vi "Rang wear off.vi"(8 "error in (no error)":errorcluster caption="错误输入（无错误）", 11 "Popup 输入":refnum<class "Popup.lvclass"> caption="DNL_LabVIEW Object in") -> (0 "error out":errorcluster caption="错误输出", 3 "Popup 输出":refnum<class "Popup.lvclass"> caption="DNL_LabVIEW Object out")   [LabVIEW 2017, in "Popup.lvclass"]
uses:
  Popup.lvclass
  Popup.lvclass/Popup.ctl
  <vilib>/Utility/Data Type/NI_Data Type.lvlib
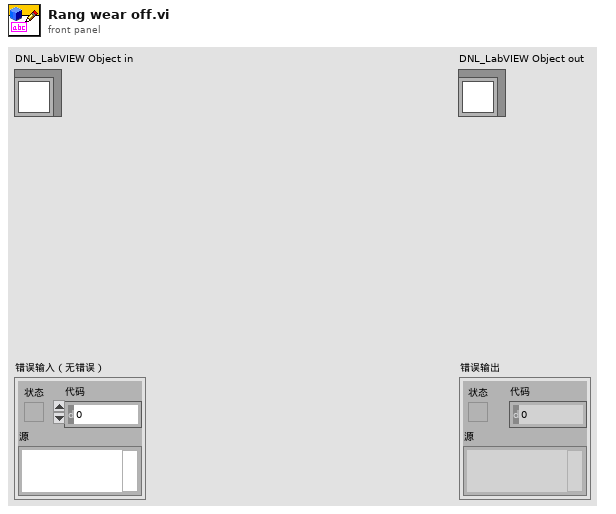
[diagram p1: front panel]
types:
  T1 = typedef "NI_Data Type.lvlib/Data Type.ctl" = enum8{"Invalid Type", "Void", "I8", "I16", "I32", "I64", "U8", "U16", "U32", "U64", "Single Float", "Double Float", "Extended Float", "Single Complex", "Double Complex", "Extended Complex", "Enum U8", "Enum U16", "Enum U32", "Enum U64", "Single Float With Unit", "Double Float With Unit", "Extended Float With Unit", "Single Complex with Unit", "Double Complex with Unit", "Extended Complex with Unit", "Boolean", "String", "Path", "Picture", "Tag", "Array", "Cluster", "Variant", "LV Variant", "Waveform", "Timestamp", "Digital Waveform", "Digital Data", "ExpressData", "Refnum", "External Data", "VI", "Poly VI", "LabVIEW Class Instance", "Fixed Point"}
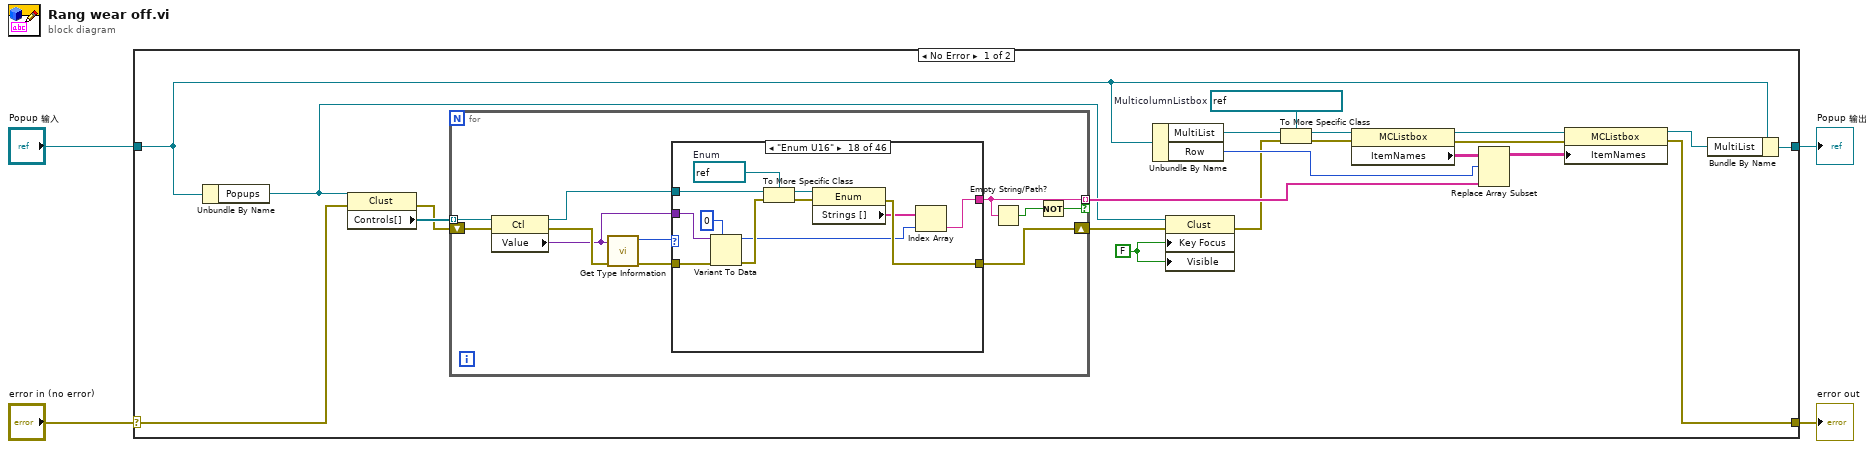
[diagram p0: block diagram]
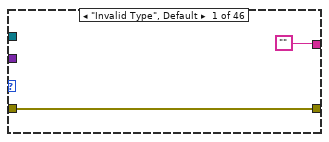
[diagram p2: hidden frame]
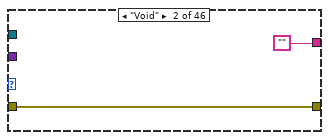
[diagram p3: hidden frame]
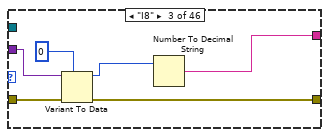
[diagram p4: hidden frame]
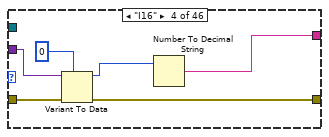
[diagram p5: hidden frame]
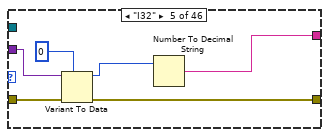
[diagram p6: hidden frame]
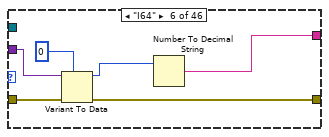
[diagram p7: hidden frame]
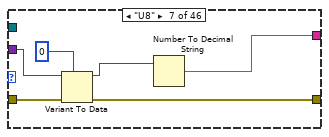
[diagram p8: hidden frame]
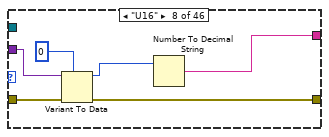
[diagram p9: hidden frame]
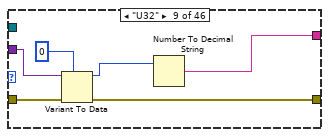
[diagram p10: hidden frame]
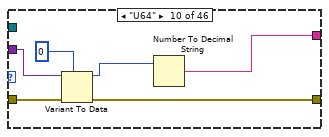
[diagram p11: hidden frame]
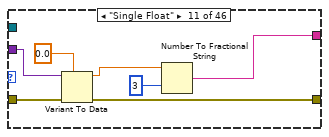
[diagram p12: hidden frame]
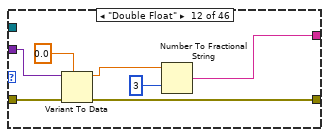
[diagram p13: hidden frame]
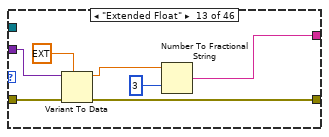
[diagram p14: hidden frame]
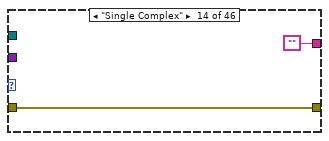
[diagram p15: hidden frame]
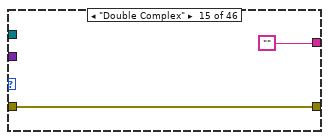
[diagram p16: hidden frame]
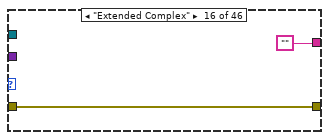
[diagram p17: hidden frame]
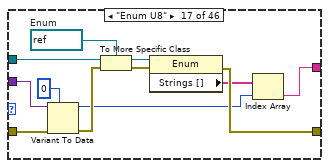
[diagram p18: hidden frame]
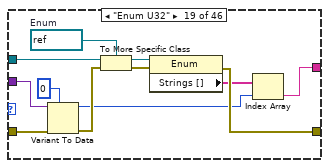
[diagram p19: hidden frame]
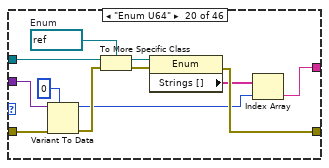
[diagram p20: hidden frame]
diagram:
  n1 = case shown="No Error" "error in (no error)" {
    selector: "error in (no error)" -> [w25 w230]
    tunnel: [w9 w230] -> w3
    tunnel: [w22 w229] -> w1
    tunnel: "Popup 输入" -> [w21 w229]
    frame No Error {
      w6 = FALSE
      w17 = refnum<vi> refnum  # MulticolumnListbox
      n2 = Unbundle By Name(w21) -> ("Popups"=w7:refnum<vi>)
      n3 = property class="Clust"(reference=w7, error in=w25) -> (error out=w23:errorcluster, "Controls[]"=w24:refnum<vi>[])  [unwired: 1 out]
      n4 = for {
        tunnel: w24 -> [w36] mode=indexing
        shift-right: [w30] -> w8
        shift-left: w23 -> [w35]
        tunnel: [w27] -> w14 mode=indexing if=w26
        n5 = property class="Ctl"(reference=w36, error in=w35) -> (reference out=w29:refnum<vi>, error out=w33:errorcluster, "Value"=w31:variant)
        n6 = call <vilib>:"Get Type Information.vi"("error in (no error)"=w33, "Variant"=w31) -> ("error out"=w32:errorcluster, "Type"=w34:T1)  [unwired: 5 in, 3 out]
        n7 = case shown="\"Enum U16\"" w34 {
          tunnel: w32 -> [w38 w40 w45 w51 w57 w63 w69 w75 w81 w87 w95 w102 w109 w111 w112 w114 w125 w137 w149 w161 w164 w166 w168 w170 w172 w174 w183 w188 w194 w196 w198 w200 w202 w204 w206 w208 w210 w212 w214 w216 w218 w220 w222 w224 w226 w228]
          tunnel: w31 -> [_ _ w46 w52 w58 w64 w70 w76 w82 w88 w94 w101 w108 _ _ _ w126 w138 w150 w162 _ _ _ _ _ _ w182 w187 w193 _ _ _ _ _ _ _ _ _ _ _ _ _ _ _ _ _]
          tunnel: [w38 w40 w43 w49 w55 w61 w67 w73 w79 w85 w92 w99 w106 w111 w112 w114 w119 w131 w143 w155 w164 w166 w168 w170 w172 w174 w176 w185 w190 w196 w198 w200 w202 w204 w206 w208 w210 w212 w214 w216 w218 w220 w222 w224 w226 w228] -> w30
          tunnel: ["" "" w41 w47 w53 w59 w65 w71 w77 w83 w89 w96 w103 "" "" "" w116 w128 w140 w152 "" "" "" "" "" "" w177 w184 w189 "" "" "" "" "" "" "" "" "" "" "" "" "" "" "" "" ""] -> w27
          tunnel: w29 -> [_ _ _ _ _ _ _ _ _ _ _ _ _ _ _ _ w127 w139 w151 w163 _ _ _ _ _ _ _ _ _ _ _ _ _ _ _ _ _ _ _ _ _ _ _ _ _ _]
          frame "Invalid Type", Default {
          }
          frame "Void" {
          }
          frame "I8" {
            n8 = Variant To Data(error in=w45, type=i8 0, Variant=w46) -> (data=w42:i8, error out=w43:errorcluster)
            n9 = Number To Decimal String(number=w42) -> (decimal integer string=w41:string)  [unwired: 1 in]
          }
          frame "I16" {
            n10 = Variant To Data(error in=w51, type=i16 0, Variant=w52) -> (data=w48:i16, error out=w49:errorcluster)
            n11 = Number To Decimal String(number=w48) -> (decimal integer string=w47:string)  [unwired: 1 in]
          }
          frame "I32" {
            n12 = Variant To Data(error in=w57, type=0, Variant=w58) -> (data=w54:i32, error out=w55:errorcluster)
            n13 = Number To Decimal String(number=w54) -> (decimal integer string=w53:string)  [unwired: 1 in]
          }
          frame "I64" {
            n14 = Variant To Data(error in=w63, type=i64 0, Variant=w64) -> (data=w60:i64, error out=w61:errorcluster)
            n15 = Number To Decimal String(number=w60) -> (decimal integer string=w59:string)  [unwired: 1 in]
          }
          frame "U8" {
            n16 = Variant To Data(error in=w69, type=u8 0, Variant=w70) -> (data=w66:u8, error out=w67:errorcluster)
            n17 = Number To Decimal String(number=w66) -> (decimal integer string=w65:string)  [unwired: 1 in]
          }
          frame "U16" {
            n18 = Variant To Data(error in=w75, type=u16 0, Variant=w76) -> (data=w72:u16, error out=w73:errorcluster)
            n19 = Number To Decimal String(number=w72) -> (decimal integer string=w71:string)  [unwired: 1 in]
          }
          frame "U32" {
            n20 = Variant To Data(error in=w81, type=u32 0, Variant=w82) -> (data=w78:u32, error out=w79:errorcluster)
            n21 = Number To Decimal String(number=w78) -> (decimal integer string=w77:string)  [unwired: 1 in]
          }
          frame "U64" {
            n22 = Variant To Data(error in=w87, type=u64 0, Variant=w88) -> (data=w84:u64, error out=w85:errorcluster)
            n23 = Number To Decimal String(number=w84) -> (decimal integer string=w83:string)  [unwired: 1 in]
          }
          frame "Single Float" {
            n24 = Variant To Data(error in=w95, type=sgl 0.0, Variant=w94) -> (data=w91:sgl, error out=w92:errorcluster)
            n25 = Number To Fractional String(number=w91, precision (6)=3) -> (F-format string=w89:string)  [unwired: 2 in]
          }
          frame "Double Float" {
            n26 = Variant To Data(error in=w102, type=0.0, Variant=w101) -> (data=w98:dbl, error out=w99:errorcluster)
            n27 = Number To Fractional String(number=w98, precision (6)=3) -> (F-format string=w96:string)  [unwired: 2 in]
          }
          frame "Extended Float" {
            n28 = Variant To Data(error in=w109, type=ext 0.0, Variant=w108) -> (data=w105:ext, error out=w106:errorcluster)
            n29 = Number To Fractional String(number=w105, precision (6)=3) -> (F-format string=w103:string)  [unwired: 2 in]
          }
          frame "Single Complex" {
          }
          frame "Double Complex" {
          }
          frame "Extended Complex" {
          }
          frame "Enum U8" {
            w122 = refnum<vi> refnum  # Enum
            n30 = Variant To Data(error in=w125, type=u8 0, Variant=w126) -> (data=w117:u8, error out=w123:errorcluster)
            n31 = To More Specific Class(target class=w122, reference=w127, error in=w123) -> (specific class reference=w121:refnum<vi>, error out=w120:errorcluster)
            n32 = property class="Enum"(reference=w121, error in=w120) -> (error out=w119:errorcluster, "Strings []"=w118:string[])  [unwired: 1 out]
            n33 = Index Array(array=w118, index=w117) -> (element=w116:string)
          }
          frame "Enum U16" {
            w134 = refnum<vi> refnum  # Enum
            n34 = Variant To Data(error in=w137, type=u16 0, Variant=w138) -> (data=w129:u16, error out=w135:errorcluster)
            n35 = To More Specific Class(target class=w134, reference=w139, error in=w135) -> (specific class reference=w133:refnum<vi>, error out=w132:errorcluster)
            n36 = property class="Enum"(reference=w133, error in=w132) -> (error out=w131:errorcluster, "Strings []"=w130:string[])  [unwired: 1 out]
            n37 = Index Array(array=w130, index=w129) -> (element=w128:string)
          }
          frame "Enum U32" {
            w146 = refnum<vi> refnum  # Enum
            n38 = Variant To Data(error in=w149, type=u32 0, Variant=w150) -> (data=w141:u32, error out=w147:errorcluster)
            n39 = To More Specific Class(target class=w146, reference=w151, error in=w147) -> (specific class reference=w145:refnum<vi>, error out=w144:errorcluster)
            n40 = property class="Enum"(reference=w145, error in=w144) -> (error out=w143:errorcluster, "Strings []"=w142:string[])  [unwired: 1 out]
            n41 = Index Array(array=w142, index=w141) -> (element=w140:string)
          }
          frame "Enum U64" {
            w158 = refnum<vi> refnum  # Enum
            n42 = Variant To Data(error in=w161, type=u64 0, Variant=w162) -> (data=w153:u64, error out=w159:errorcluster)
            n43 = To More Specific Class(target class=w158, reference=w163, error in=w159) -> (specific class reference=w157:refnum<vi>, error out=w156:errorcluster)
            n44 = property class="Enum"(reference=w157, error in=w156) -> (error out=w155:errorcluster, "Strings []"=w154:string[])  [unwired: 1 out]
            n45 = Index Array(array=w154, index=w153) -> (element=w152:string)
          }
          frame "Single Float With Unit" {
          }
          frame "Double Float With Unit" {
          }
          frame "Extended Float With Unit" {
          }
          frame "Single Complex with Unit" {
          }
          frame "Double Complex with Unit" {
          }
          frame "Extended Complex with Unit" {
          }
          frame "Boolean" {
            n46 = Variant To Data(error in=w183, type=FALSE, Variant=w182) -> (data=w180:bool, error out=w176:errorcluster)
            n47 = Select(t="TURE", s=w180, f="FALES") -> (s? t:f=w177:string)
          }
          frame "String" {
            n48 = Variant To Data(error in=w188, type="", Variant=w187) -> (data=w184:string, error out=w185:errorcluster)
          }
          frame "Path" {
            n49 = Variant To Data(error in=w194, type=path "", Variant=w193) -> (data=w191:path, error out=w190:errorcluster)
            n50 = Path To String(path=w191) -> (string=w189:string)
          }
          frame "Picture" {
          }
          frame "Tag" {
          }
          frame "Array" {
          }
          frame "Cluster" {
          }
          frame "Variant" {
          }
          frame "LV Variant" {
          }
          frame "Waveform" {
          }
          frame "Timestamp" {
          }
          frame "Digital Waveform" {
          }
          frame "Digital Data" {
          }
          frame "ExpressData" {
          }
          frame "Refnum" {
          }
          frame "External Data" {
          }
          frame "VI" {
          }
          frame "Poly VI" {
          }
          frame "LabVIEW Class Instance" {
          }
          frame "Fixed Point" {
          }
        }
        n51 = Empty String/Path?(string/path=w27) -> (empty?=w28:bool)
        n52 = Not(x=w28) -> (.not. x?=w26:bool)
      }
      n53 = Unbundle By Name(w21) -> ("MultiList"=w20:refnum<vi>, "Row"=w15:u16)
      n54 = property class="Clust"(reference=w7, error in=w8, "Key Focus"=w6, "Visible"=w6) -> (error out=w5:errorcluster)  [unwired: 1 out]
      n55 = To More Specific Class(target class=w17, reference=w20, error in=w5) -> (specific class reference=w19:refnum<vi>, error out=w18:errorcluster)
      n56 = property class="MCListbox"(reference=w19, error in=w18) -> (reference out=w12:refnum<vi>, error out=w11:errorcluster, "ItemNames"=w16:string[][])
      n57 = Replace Array Subset(array=w16, new element=w14, index (row)=w15) -> (w13:string[][])  [unwired: 1 in]
      n58 = property class="MCListbox"(reference=w12, error in=w11, "ItemNames"=w13) -> (reference out=w10:refnum<vi>, error out=w9:errorcluster)
      n59 = Bundle By Name(cluster=w21, "MultiList"=w10) -> (w22:refnum<class "Popup.lvclass">)
    }
    frame Error {
    }
  }
  "error out" <- w3
  "Popup 输出" <- w1
